vi "Boiler Controller.vi"(8 "error in":errorcluster, 10 "Notifiers":T1, 11 "Message Queues":T2) -> (0 "error out":errorcluster)   [LabVIEW 2022 SP3]
uses:
  support/Message Queue/All Message Queues.ctl
  support/Message Queue/Message Cluster.ctl
  support/Notifiers/Notifiers.ctl
  support/Message Queue/Message Queue.lvlib
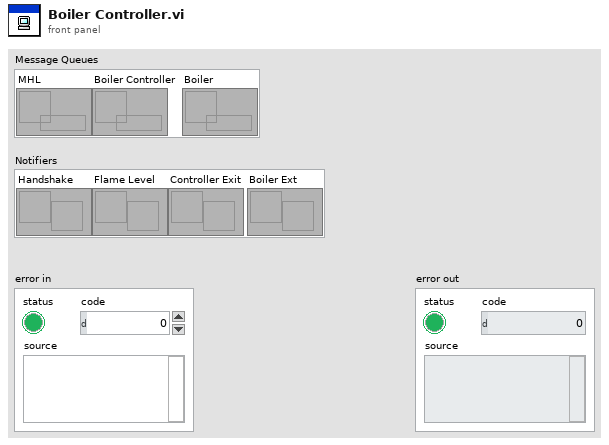
[diagram p1: front panel]
types:
  T1 = typedef "Notifiers.ctl" = cluster{"Handshake":refnum<notifier>, "Flame Level":refnum<notifier>, "Controller Exit":refnum<notifier>, "Boiler Ext":refnum<notifier>}
  T2 = typedef "Message Queue.lvlib/All Message Queues.ctl" = cluster{"MHL":refnum<queue>, "Boiler Controller":refnum<queue>, "Boiler":refnum<queue>}
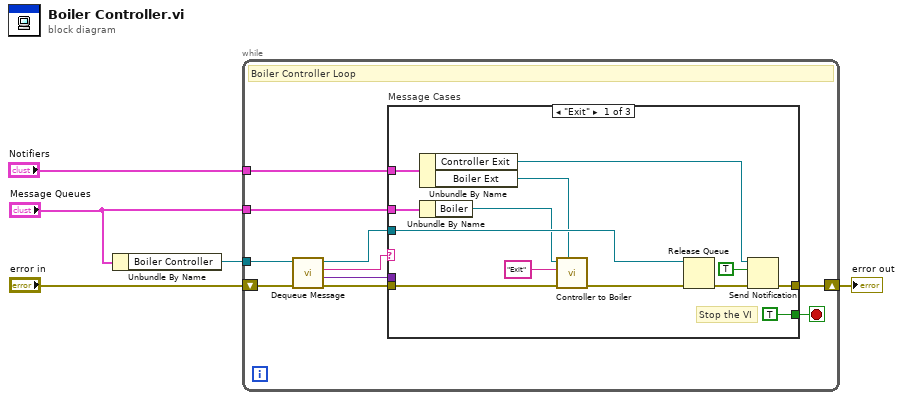
[diagram p0: block diagram]
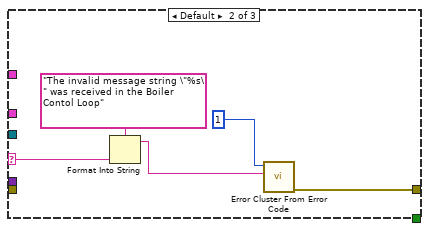
[diagram p2: hidden frame]
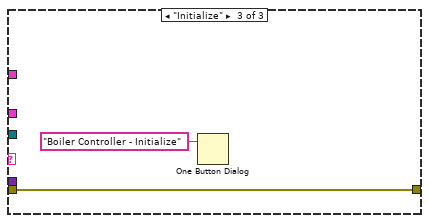
[diagram p3: hidden frame]
diagram:
  n1 = Unbundle By Name("Message Queues") -> ("Boiler Controller"=w5:refnum<queue>)
  n2 = while {
    tunnel: w5 -> [w15]
    shift-right: [w9] -> w3
    shift-left: "error in" -> [w10]
    tunnel: "Notifiers" -> [w7]
    tunnel: "Message Queues" -> [w6]
    stop <- w8 stop-if-true
    # "Boiler Controller Loop"
    n3 = call "Dequeue Message.vi"("error in"=w10, "Message Queue"=w15) -> ("error out"=w11:errorcluster, "Message Data"=w12:variant, "Message"=w14:string, "dup Message Queue"=w13:refnum<queue>)  [unwired: 6 in]
    n4 = case "Message Cases" shown="\"Exit\"" w14 {
      selector: w14 -> [_ w33 _]
      tunnel: w13 -> [w28 _ _]
      tunnel: w12 -> [_ _ _]
      tunnel: w11 -> [w25 _ w34]
      tunnel: [w18 w31 w34] -> w9
      tunnel: [TRUE _ _] -> w8
      tunnel: w7 -> [w26 _ _]
      tunnel: w6 -> [w23 _ _]
      frame "Exit" {
        # "Stop the VI"
        n5 = Unbundle By Name(w26) -> ("Controller Exit"=w17:refnum<notifier>, "Boiler Ext"=w20:refnum<notifier>)
        n6 = Unbundle By Name(w23) -> ("Boiler"=w22:refnum<queue>)
        n7 = call "Controller to Boiler.vi"("Notifier"=w20, "error in"=w25, "Message"="Exit", "Boiler Queue in"=w22) -> ("error out"=w24:errorcluster)  [unwired: 5 in, 2 out]
        n8 = Release Queue(queue=w28, error in (no error)=w24) -> (error out=w19:errorcluster)  [unwired: 1 in, 2 out]
        n9 = Send Notification(notification=TRUE, notifier=w17, error in (no error)=w19) -> (error out=w18:errorcluster)  [unwired: 1 out]
      }
      frame Default {
        n10 = Format Into String(format string="The invalid message string \"%s\" was received in the Boiler Contol Loop", w33) -> (resulting string=w30:string)  [unwired: 2 in, 1 out]
        n11 = call <vilib>:"Error Cluster From Error Code.vi"("error message (\"\")"=w30, "error code (0)"=1) -> ("error out"=w31:errorcluster)  [unwired: 7 in]
      }
      frame "Initialize" {
        n12 = One Button Dialog(message="Boiler Controller - Initialize") -> ()  [unwired: 1 in, 1 out]
      }
    }
  }
  "error out" <- w3
